vi "qVOL.vi"(0 "System no.":i32=1 min=1 max=4 step=1, 2 "Axes to query":string[](array[string]), 3 "All axes?":bool, 4 "Axis identifier?":bool=TRUE, 5 "error in":errorcluster) -> (14 "Current PZT voltage":dbl[](array[numeric]) format="%.6f", 15 "Channels to query out":string[](array[string]), 19 "error out":errorcluster)   [LabVIEW 2026]
doc: "Returns current PZT voltage for queried axes / piezo channels.\n\nAnalog: If All axes? = TRUE, then Axis identifier? can be FALSE. VI reads control voltage.\n\nE-516: If All axes? = TRUE, then Axis identifier? must be TRUE\n\nE-710: If All axes? = TRUE, then Axis identifier? must be TRUE. Axes to query are piezo channel numbers.\n\nC-413, E-517, E-518, E-709, E-712, E-725, E-727, E-753, E-754, E-755: If All axes? = TRUE, then Axis identifier? can be FALSE. Axes to query are piezo channel numbers.\n\nE-761: If All axes? = TRUE, then Axis identifier? can be FALSE. Axes to query are piezo channel numbers, which can be 1 to 4.\n\nE-816: All axes? = FALSE, only one axis per command allowed."
panel:
  # "Returns current PZT voltage for queried axes / piezo channels."
  # "If all axes: use"
  # "Query"
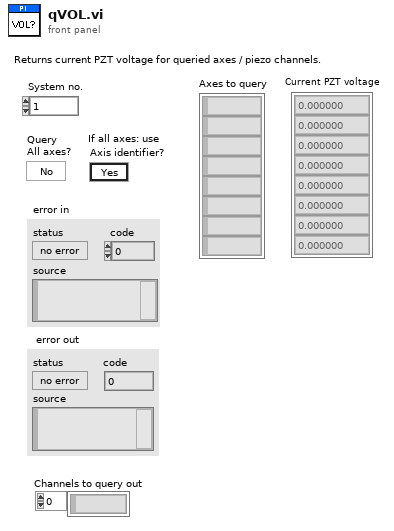
[diagram p1: front panel]
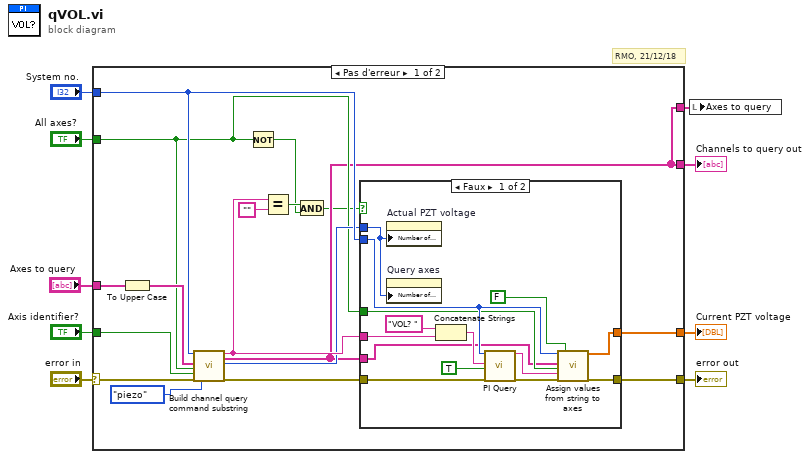
[diagram p0: block diagram]
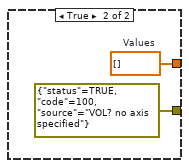
[diagram p2: hidden frame]
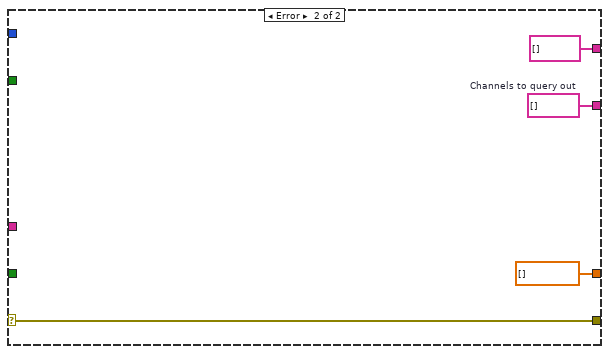
[diagram p3: hidden frame]
diagram:
  # "RMO, 21/12/18"
  n1 = case shown="Pas d'erreur" "error in" {
    selector: "error in" -> [w10 w44]
    tunnel: [w26 dbl[] [] ("Values")] -> w9
    tunnel: "Axes to query" -> [w25 _]
    tunnel: [w13 w44] -> w7
    tunnel: "Axis identifier?" -> [w15 _]
    tunnel: "System no." -> [w19 _]
    tunnel: [w12 string[] [] ("Axes to query out")] -> w4
    tunnel: "All axes?" -> [w14 _]
    tunnel: [w12 w43] -> w2
    frame No Error {
      n2 = To Upper Case(1:w25) -> (0:w16:string[])
      n3 = call "Build channel query command substring.vi"("System no."=w19, "Channels to query in"=w16, "Query\nAll channels?"=w14, "For all channels: use\nChannel identifier?"=w15, "error in"=w10, "Channel type"=enum16{"piezo", "sensor"}."piezo") -> ("Command substring"=w18:string, "Channels to query out"=w12:string[], "Number of rows"=w17:u32, "error out"=w20:errorcluster)  [unwired: 1 in, 9 out]
      n4 = Not(x=w14) -> (.not. x?=w22:bool)
      n5 = Equal?(x=w18, y="" ("x")) -> (x = y?=w23:bool)
      n6 = And(x=w23, y=w22) -> (x .and. y?=w11:bool)
      n7 = case shown="Faux" w11 {
        tunnel: [w37 w41] -> w26
        tunnel: w20 -> [w36 _]
        tunnel: w19 -> [w35 _]
        tunnel: w18 -> [w34 _]
        tunnel: w17 -> [w33 _]
        tunnel: w14 -> [w31 _]
        tunnel: [w30 errorcluster {"status"=TRUE, "code"=100, "source"="VOL? no axis specified"} ("error out")] -> w13
        tunnel: w12 -> [w29 _]
        frame False {
          n8 = property on="Actual PZT voltage" class="Tabl (strict)"("Number of Rows"=w33) -> ()  [unwired: 2 in, 2 out]
          n9 = property on="Query axes" class="Tabl (strict)"("Number of Rows"=w33) -> ()  [unwired: 2 in, 2 out]
          n10 = Concatenate Strings("VOL? ", w34) -> (w38:string)
          n11 = call "PI Query.vi"("System no."=w35, "String to send"=w38, "Attach termination char.?"=TRUE ("Attach Linefeed?"), "error in"=w36) -> ("String read"=w27:string, "error out"=w28:errorcluster)  [unwired: 3 in, 11 out]
          n12 = call "Assign values from string to axes.vi"("System no."=w35, "Queried axes"=w29, "All axes queried?"=w31, "Input String"=w27, "error in"=w28, "Axes related?"=FALSE) -> ("Values"=w37:dbl[], "error out"=w30:errorcluster)  [unwired: 3 in, 9 out]
        }
        frame True {
          w41 = dbl[] []  # Values
        }
      }
    }
    frame Error {
      w43 = string[] []  # Channels to query out
    }
  }
  "error out" <- w7
  "Current PZT voltage" <- w9
  "Channels to query out" <- w2
  n13 = local write "Axes to query"(w4) -> ()
